vi "Esboco.vi"() -> ()   [LabVIEW 2016]
panel:
  in  "END":bool
  out "Porta Serial":string
  out "Velocidade Real":dbl
  in  "Write":bool
  in  "Velocidade Desejada":dbl
  out "Waveform Graph":dbl[](graph)
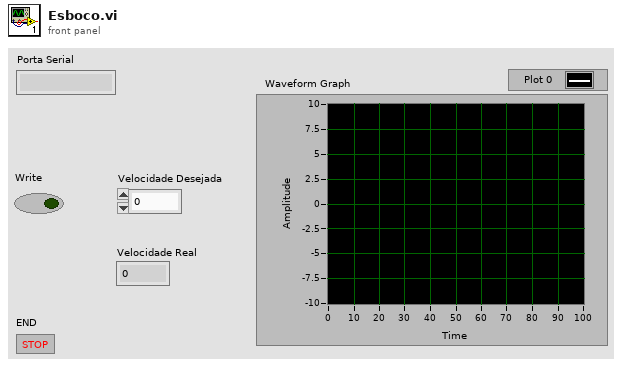
[diagram p1: front panel]
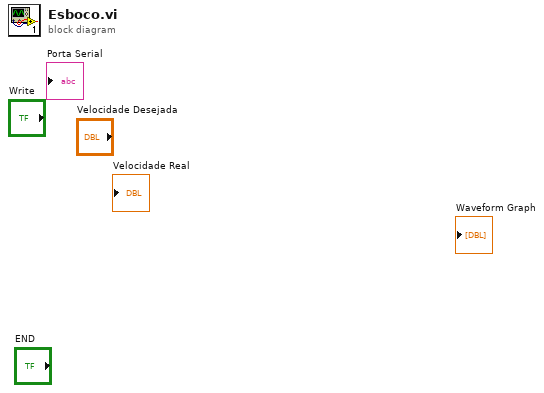
[diagram p0: block diagram]
diagram:
